vi "check_fault.vi"(4 "Reset":bool, 6 "Parameters":T1={"Stimulus"={"Type"=enum."Off", "Delay"=0, "Amplitude"=[0.0, 0.0, 0.0], "Injection point"=enum."Total pose", "Closed loop"=FALSE, "Offset"=[0.0, 0.0, 0.0], "Tip -> world"=TRUE}, "Goal Filter A"={"Lower Fc"=0.0, "Lower Q"=0.15, "Scale factor"=0.0, "Upper Fc"=0.0075, "Upper Q"=0.01, "Manip zeroing"=0.001, "Speedup max"=150.0, "Speedup thresh"=5.0, "Speedup nonlin"=3.0, "V limit"=300.0, "V limit range"=300.0}, "Mode controls"={"Hold"=FALSE, "Cancellation"=FALSE, "Goal filter"=FALSE, "Trigger"=FALSE}, "Manipulator type"=enum."Current piezo", "Manipulator calibration"={"Inverse Kinematics"=[[-0.4736411481566654, -0.25724305819165183, -1.1087933259307599], [0.296735958809338, -0.258643951607561, -1.0971603505753995], [-0.043664688535758014, 0.44635679599468125, -1.1035515399424176]], "Handle transform"=[[3.281333089700394, 0.23462731743748497, 0.17832137948371765, -8265.081657965618], [-0.20249098046098263, 2.6933210343964133, -0.2815002765708058, -33565.66155248382], [-0.14581170473284072, 0.6821648518522063, 0.8833544952169589, 26862.18782130476], [-1.1202010727438122e-18, 5.861467994999758e-19, 1.760134464394436e-18, 0.999999999999992]], "Tip offset"=[0.0, 0.0, 36200.0], "Probe calibration"=[], "Pivot position"=[0.0, 0.0, -11360.0], "Axial filter"={"filter structure"=enum."IIR 2nd Order", "Reverse Coefficients"=[0.0, 0.0], "Forward Coefficients"=[1.0, 0.0, 0.0]}, "Lateral filter"={"filter structure"=enum."IIR 2nd Order", "Reverse Coefficients"=[0.0, 0.0], "Forward Coefficients"=[1.0, 0.0, 0.0]}}, "Charge piezo"={"Capacitance"=4e-08, "V min"=-235.0, "V max"=50.0, "- margin"=465.0, "+ margin"=0.001, "I max"=40000.0, "I sat"=90000000.0, "R series"=5.0, "R shunt"=1000.0, "Fault V"=0.0, "Start Fault V"=0.0, "Start Cycles"=0, "Prop gain"=1e-06, "Int gain"=0.0, "Diff gain"=0.0}, "Network"={"Remote Host"="192.168.1.3", "Send Status"=TRUE, "Send Port"=50, "Recv Commands"=FALSE, "Recv Port"=0}, "Goal Filter B"={"Lower Fc"=1.0, "Lower Q"=2.0, "Scale factor"=61557.0, "Upper Fc"=20.0, "Upper Q"=61557.0, "Manip zeroing"=2.0, "Speedup max"=1.0, "Speedup thresh"=300.0, "Speedup nonlin"=3.0, "V limit"=300.0, "V limit range"=300.0}, "Cancellation"={"Bandwidth"=0.0, "Delay"=0, "Stack travel"=0.0, "Saturation pos"=0.0075, "Slew Limit"=0.01, "Turnoff zeroing"=0.001, "Bypass"=FALSE}, "Transition time"=3.0} {"Transition time" format="%_3f"; "Cancellation"."Slew Limit" format="%#_3p"; "Cancellation"."Saturation pos" format="%#.1f"; "Cancellation"."Stack travel" format="%#.1f"; "Cancellation"."Turnoff zeroing" format="%#_6e"; "Cancellation"."Delay" step=1; "Cancellation"."Bandwidth" min=10 max=1000 step=10; "Goal Filter B"."V limit range" format="%_3p"; "Goal Filter B"."V limit" format="%_3p"; "Goal Filter B"."Speedup nonlin" format="%_3p"; "Goal Filter B"."Upper Q" format="%_3f"; "Goal Filter B"."Upper Fc" format="%_3p"; "Goal Filter B"."Lower Q" format="%_3f"; "Goal Filter B"."Speedup thresh" format="%_3p"; "Goal Filter B"."Speedup max" format="%_3p"; "Goal Filter B"."Manip zeroing" format="%_3p"; "Goal Filter B"."Scale factor" format="%_3f"; "Goal Filter B"."Lower Fc" format="%_3p"; "Charge piezo"."I sat" format="%#_6p"; "Charge piezo"."+ margin" format="%#_6p"; "Charge piezo"."- margin" format="%#_6p"; "Charge piezo"."Start Fault V" format="%#_6p"; "Charge piezo"."R shunt" format="%#_6p"; "Charge piezo"."Prop gain" format="%#_6p"; "Charge piezo"."Fault V" format="%#_6p"; "Charge piezo"."I max" format="%#_6p"; "Charge piezo"."Diff gain" format="%#_6p"; "Charge piezo"."Int gain" format="%#_6p"; "Charge piezo"."R series" format="%#_6p"; "Charge piezo"."Capacitance" format="%#_6p"; "Manipulator calibration"."Probe calibration" format="%#.1f"; "Manipulator calibration"."Handle transform" format="%#_3f"; "Manipulator calibration"."Inverse Kinematics" format="%#_3f"; "Goal Filter A"."V limit range" format="%_3p"; "Goal Filter A"."V limit" format="%_3p"; "Goal Filter A"."Speedup nonlin" format="%_3p"; "Goal Filter A"."Upper Q" format="%_3f"; "Goal Filter A"."Upper Fc" format="%_3p"; "Goal Filter A"."Lower Q" format="%_3f"; "Goal Filter A"."Speedup thresh" format="%_3p"; "Goal Filter A"."Speedup max" format="%_3p"; "Goal Filter A"."Manip zeroing" format="%_3p"; "Goal Filter A"."Scale factor" format="%_3f"; "Goal Filter A"."Lower Fc" format="%_3p"; "Stimulus"."Offset" step=100; "Stimulus"."Amplitude" step=100; "Stimulus"."Delay" step=100}, 8 "V error":sgl[](array[numeric]), 9 "Integrator saturation":bool, 10 "I in":sgl[](array[numeric])) -> (0 "Startup over":bool, 2 "I out":sgl[](array[numeric]))   [LabVIEW 2010]
uses:
  testing/Micron params.ctl
  testing/stimulus.ctl
  testing/injection_point.ctl
  filtering/goal_filter_parms.ctl
  testing/mode_conrols.ctl
  testing/manipulator_cal.ctl
  <vilib>/Analysis/Matrix/Datatypes/RealMatrix.ctl
  asap/labview/testing/probe_calibration.ctl
  Charge controller params.ctl
  host/network_params.ctl
  cancellation/im_control_params.ctl
  <vilib>/Analysis/Matrix/NI_Matrix.lvlib
panel:
  in  "Startup counter":i32
  # "Locals:"
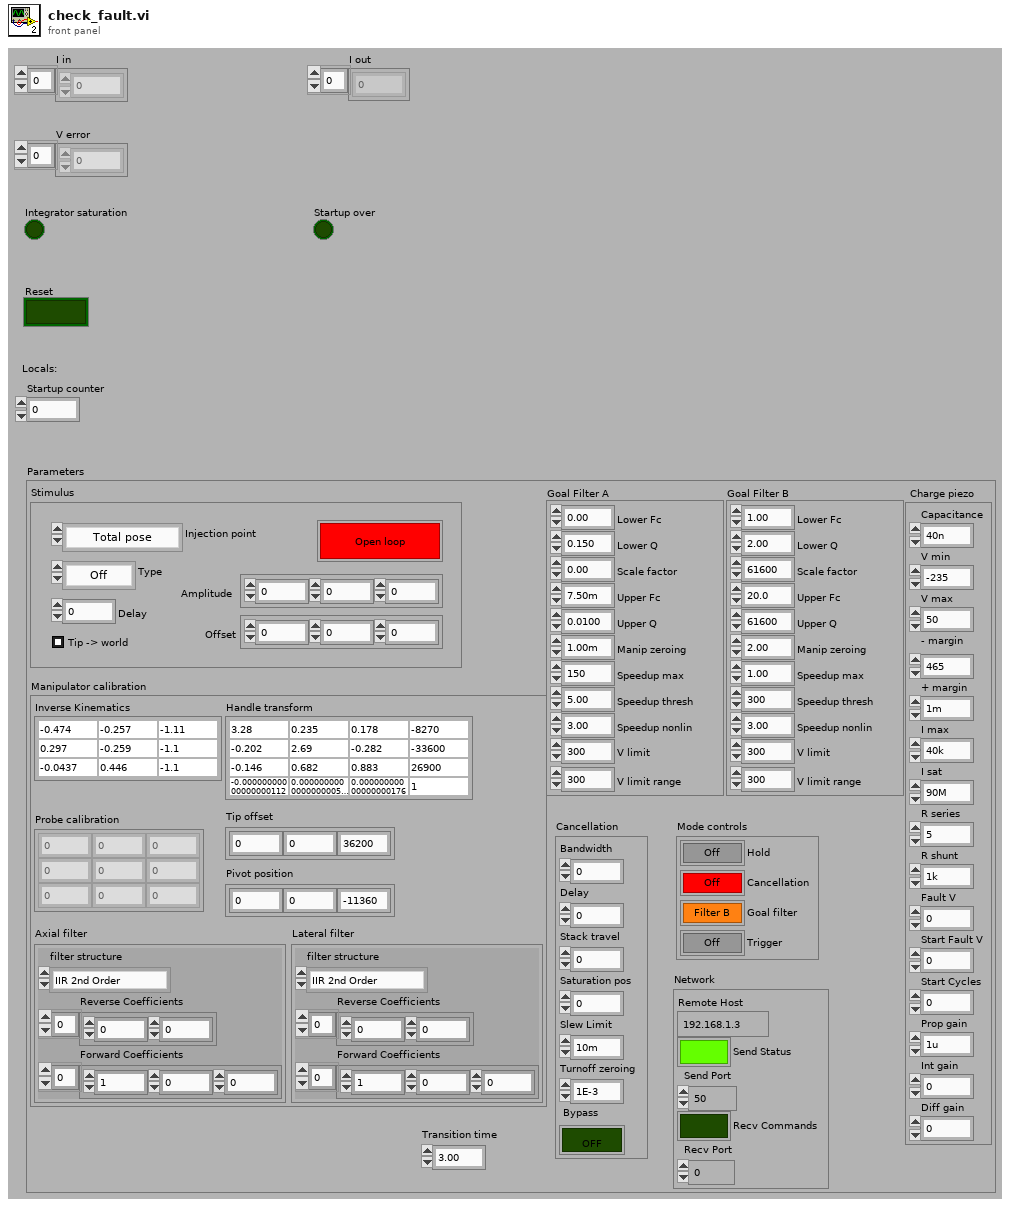
[diagram p1: front panel]
types:
  T1 = typedef "Micron params.ctl" = cluster{"Stimulus":T2, "Goal Filter A":T4, "Mode controls":T5, "Manipulator type":enum16{"Current piezo", "Voltage piezo"}, "Manipulator calibration":T6, "Charge piezo":T9, "Network":T10, "Goal Filter B":T4, "Cancellation":T11, "Transition time":sgl}
  T2 = typedef "stimulus.ctl" = cluster{"Type":enum16{"Off", "Step", "Sine", "Triangle", "Arbitrary"}, "Delay":i32, "Amplitude":sgl[], "Injection point":T3, "Closed loop":bool, "Offset":sgl[], "Tip -> world":bool}
  T3 = typedef "injection_point.ctl" = enum16{"Total pose", "V limiter", "Goal position", "Tip error (manip)", "Inverse kin", "Controller", "Stack position", "Stack drive", "DAC"}
  T4 = typedef "goal_filter_parms.ctl" = cluster{"Lower Fc":sgl, "Lower Q":sgl, "Scale factor":sgl, "Upper Fc":sgl, "Upper Q":sgl, "Manip zeroing":sgl, "Speedup max":sgl, "Speedup thresh":sgl, "Speedup nonlin":sgl, "V limit":sgl, "V limit range":sgl}
  T5 = typedef "mode_conrols.ctl" = cluster{"Hold":bool, "Cancellation":bool, "Goal filter":bool, "Trigger":bool}
  T6 = typedef "manipulator_cal.ctl" = cluster{"Inverse Kinematics":T7, "Handle transform":T7, "Tip offset":sgl[], "Probe calibration":T8, "Pivot position":sgl[], "Axial filter":cluster{"filter structure":enum32{"IIR 2nd Order", "IIR 4th Order"}, "Reverse Coefficients":dbl[], "Forward Coefficients":dbl[]}, "Lateral filter":cluster{"filter structure":enum32{"IIR 2nd Order", "IIR 4th Order"}, "Reverse Coefficients":dbl[], "Forward Coefficients":dbl[]}}
  T7 = typedef "NI_Matrix.lvlib/RealMatrix.ctl" = dbl[][]
  T8 = typedef "probe_calibration.ctl" = sgl[][]
  T9 = typedef "Charge controller params.ctl" = cluster{"Capacitance":sgl, "V min":sgl, "V max":sgl, "- margin":sgl, "+ margin":sgl, "I max":sgl, "I sat":sgl, "R series":sgl, "R shunt":sgl, "Fault V":sgl, "Start Fault V":sgl, "Start Cycles":i32, "Prop gain":sgl, "Int gain":sgl, "Diff gain":sgl}
  T10 = typedef "network_params.ctl" = cluster{"Remote Host":string, "Send Status":bool, "Send Port":u16, "Recv Commands":bool, "Recv Port":u16}
  T11 = typedef "im_control_params.ctl" = cluster{"Bandwidth":sgl, "Delay":i32, "Stack travel":sgl, "Saturation pos":sgl, "Slew Limit":sgl, "Turnoff zeroing":sgl, "Bypass":bool}
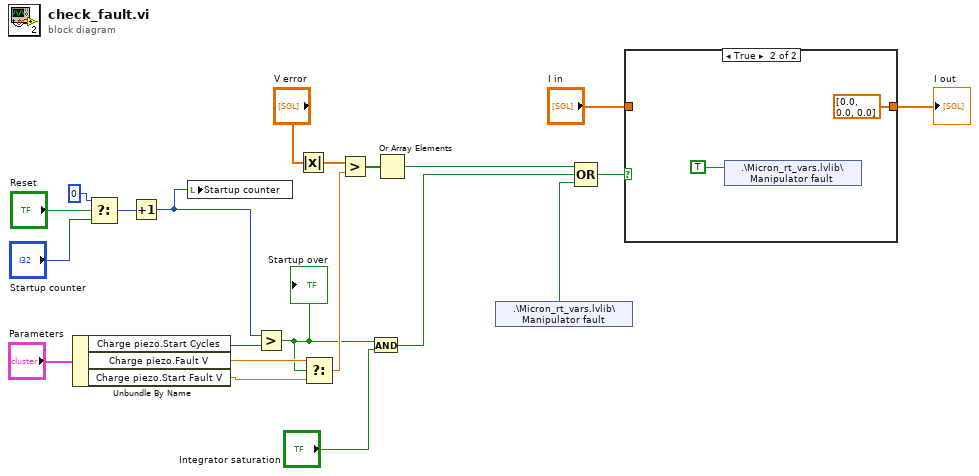
[diagram p0: block diagram]
diagram:
  n1 = Unbundle By Name("Parameters") -> ("Charge piezo.Start Cycles"=w9:i32, "Charge piezo.Fault V"=w8:sgl, "Charge piezo.Start Fault V"=w7:sgl)
  n2 = Select(t=0, s="Reset", f="Startup counter") -> (s? t:f=w10:i32)
  n3 = Increment(x=w10) -> (x+1=w5:i32)
  n4 = local write "Startup counter"(w5) -> ()
  n5 = Greater?(x=w5, y=w9) -> (0:w4:bool)
  "Startup over" <- w4
  n6 = Absolute Value(x="V error") -> (abs(x)=w21:sgl[])
  n7 = Select(t=w8, s=w4, f=w7) -> (s? t:f=w6:sgl)
  n8 = Greater?(x=w21, y=w6) -> (0:w19:bool[])
  n9 = And(x=w4, y="Integrator saturation") -> (x .and. y?=w2:bool)
  n10 = Or Array Elements(Boolean array=w19) -> (logical OR=w18:bool)
  n11 = shared-variable ".\\Micron_rt_vars.lvlib\\Manipulator fault"() -> (w17:bool)  [unwired: 2 out]
  n12 = Compound Arithmetic op=OR(w18, w2, w17) -> (w1:bool)
  n13 = case shown="True" w1 {
    tunnel: [w22 sgl[] [0.0, 0.0, 0.0] ("I in")] -> w15
    tunnel: "I in" -> [w22 _]
    frame False {
    }
    frame True {
      n14 = shared-variable ".\\Micron_rt_vars.lvlib\\Manipulator fault"(TRUE ("Manipulator fault")) -> ()  [unwired: 2 out]
    }
  }
  "I out" <- w15
